vi "CDAQ Configuration.vi"(8 "error in (no error)":errorcluster, 11 "Configuration in":refnum<class "Configuration.lvclass">) -> (0 "error out":errorcluster, 3 "Configuration out":refnum<class "Configuration.lvclass">)   [LabVIEW 2017, in "CompactDAQ Configuration.lvclass"]
uses:
  CompactDAQ Configuration.lvclass
  <userlib>/Configuration Dialog Actor/Configuration.lvclass
  \\Mac\Home/Documents/Extensible-Config-Dialog/Configuration.lvclass
  CompactDAQ Configuration.lvclass/CompactDAQ Configuration.ctl
panel:
  in  "CompactDAQ Settings":cluster{"Allow Muxing?":bool}
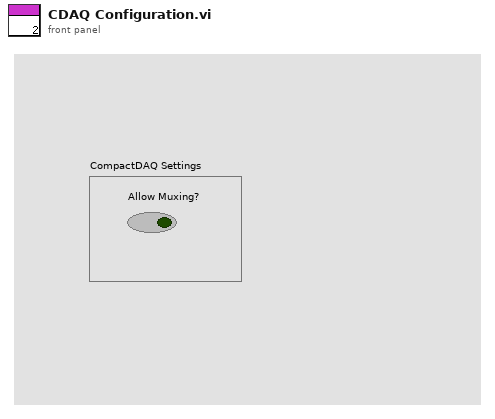
[diagram p1: front panel]
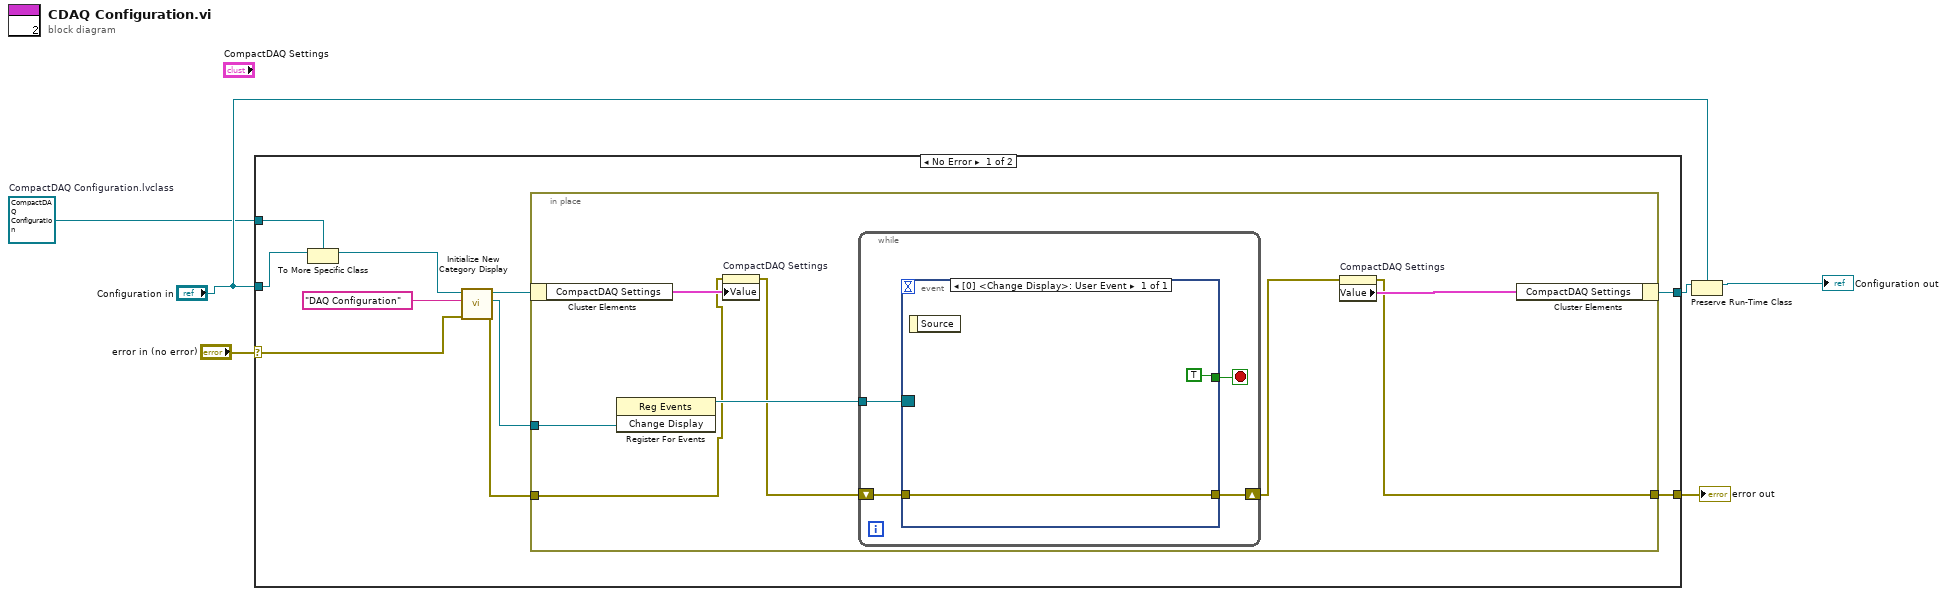
[diagram p0: block diagram]
diagram:
  w1 = refnum<class "CompactDAQ Configuration.lvclass"> refnum  # CompactDAQ Configuration.lvclass
  n1 = case shown="No Error" "error in (no error)" {
    selector: "error in (no error)" -> [w13 w32]
    tunnel: [w12 w31] -> w3
    tunnel: [w7 w32] -> w6
    tunnel: "Configuration in" -> [w11 w31]
    tunnel: w1 -> [w9 _]
    frame No Error {
      n2 = To More Specific Class(target class=w9, reference=w11) -> (specific class reference=w10:refnum<class "CompactDAQ Configuration.lvclass">)  [unwired: 1 in, 1 out]
      n3 = call <userlib>:"Initialize New Category Display.vi"("error in (no error)"=w13, "Name to Display"="DAQ Configuration", "Configuration in"=w10) -> ("error out"=w15:errorcluster, "Change Display"=w16:refnum<user-event>, "Configuration Out"=w8:refnum<class "CompactDAQ Configuration.lvclass">)  [unwired: 6 in]
      n4 = in-place {
        in-place-border: w16 -> [w24]
        in-place-border: w15 -> [w20]
        in-place-border: [w17] -> w7
        n5 = in-place-cluster #1(w8) -> ("CompactDAQ Settings"=w22:cluster{"Allow Muxing?":bool})
        n6 = register-events(w24) -> (reference out=w23:refnum<event-registration>)  [unwired: 2 in, 1 out]
        n7 = property on="CompactDAQ Settings" class="Clust (strict)"(error in=w20, "Value"=w22) -> (error out=w21:errorcluster)  [unwired: 1 in, 1 out]
        n8 = while {
          tunnel: w23 -> [w27]
          shift-right: [w26] -> w18
          shift-left: w21 -> [w25]
          stop <- w28 stop-if-true
          n9 = event shown="[0] <Change Display>: User Event" {
            selector: w27 -> [_]
            dyn-events: _ -> [_]
            timeout: _ -> [_]
            tunnel: [TRUE] -> w28
            tunnel: [w29] -> w26
            tunnel: w25 -> [w29]
            event User Event {
              n10 = event-data() -> ()  [unwired: 1 in, 1 out]
            }
          }
        }
        n11 = property on="CompactDAQ Settings" class="Clust (strict)"(error in=w18) -> (error out=w17:errorcluster, "Value"=w19:cluster{"Allow Muxing?":bool})  [unwired: 1 in, 1 out]
        n12 = in-place-cluster #1("CompactDAQ Settings"=w19) -> (w12:refnum<class "CompactDAQ Configuration.lvclass">)
      }
    }
    frame Error {
    }
  }
  "error out" <- w6
  n13 = Preserve Run-Time Class(object in=w3, 2:"Configuration in") -> (object out=→"Configuration out":refnum<class "Configuration.lvclass">)  [unwired: 1 in, 1 out]
